vi "Data_DisplayMode.vi"(0 "taskHandle":variant, 1 "显示方式":u16(ring) items=["原始显示", "拆分显示"], 5 "1D data":dbl[](array[numeric]), 7 "displayLength":u32, 9 "wfm info":T1, 11 "error in":errorcluster) -> (4 "task handle":variant, 10 "2D data":dbl[][](array[numeric]), 15 "error out":errorcluster)   [LabVIEW 2013]
uses:
  <userlib>/ArtScope/_SubVI/ArtScope_ArrayByChannel_DBL.vi
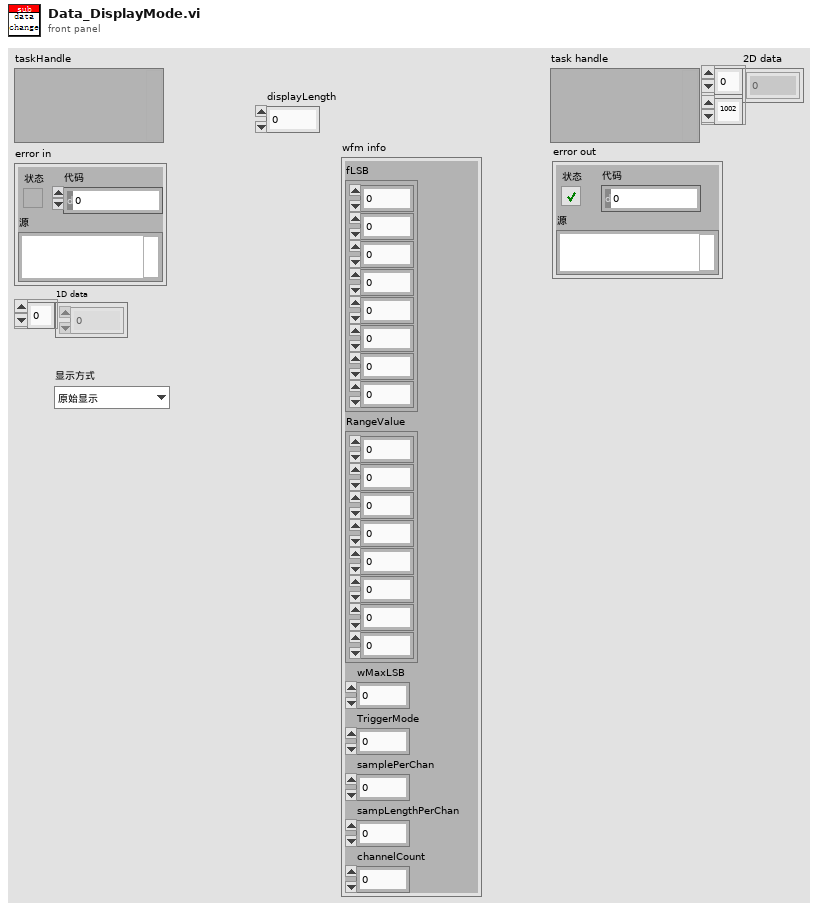
[diagram p1: front panel]
types:
  T1 = cluster{"fLSB":cluster{dbl, dbl, dbl, dbl, dbl, dbl, dbl, dbl}, "RangeValue":cluster{dbl, dbl, dbl, dbl, dbl, dbl, dbl, dbl}, "wMaxLSB":u32, "TriggerMode":i32, "samplePerChan":u32, "sampLengthPerChan":u32, "channelCount":i32}
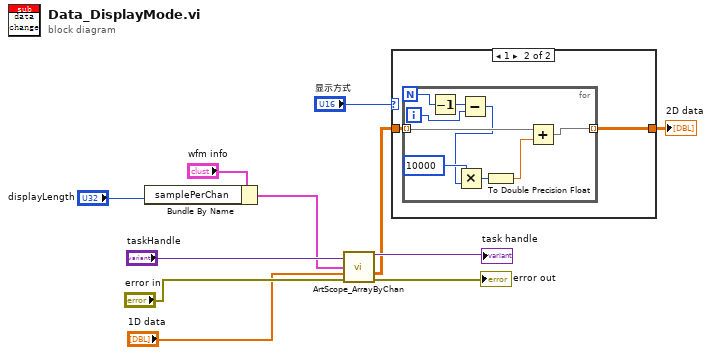
[diagram p0: block diagram]
diagram:
  n1 = Bundle By Name(cluster="wfm info", "samplePerChan"="displayLength") -> (w6:T1)
  n2 = call-poly <userlib>:"ArtScope_ArrayByChan.vi"("task handle"="taskHandle", "wfm info"=w6, "1D data"="1D data", "error in (no error)"="error in") -> ("task handle"=→"task handle":variant, "2D data"=w3:dbl[][], "error out"=→"error out":errorcluster)  [unwired: 9 in]
  n3 = case shown="1" "显示方式" {
    tunnel: w3 -> [w12 w14]
    tunnel: [w12 w13] -> w1
    frame 0, Default {
    }
    frame 1 {
      n4 = for {
        N -> [w18]
        tunnel: w14 -> [w23] mode=indexing
        tunnel: [w19] -> w13 mode=indexing
        i -> [w16]
        n5 = Decrement(x=w18) -> (x-1=w17:i32)
        n6 = Subtract(x=w17, y=w16) -> (x-y=w15:i32)
        n7 = Multiply(x=10000, y=w15) -> (x*y=w21:i32)
        n8 = To Double Precision Float(number=w21) -> (double precision float=w20:dbl)
        n9 = Add(x=w23, y=w20) -> (x+y=w19:dbl[])
      }
    }
  }
  "2D data" <- w1
